vi "Conversion_from_SI_units.vi"(6 "Microsteps (MS=64)":dbl, 7 "Motor":u16(ring) items=["none", "1", "2", "3", "4", "all"], 8 "Output Unit":T1=enum."Meter", 10 "Input":dbl) -> (2 "Output":dbl)   [LabVIEW 2013]
uses:
  ConversionAndInformation/Unit_Control.ctl
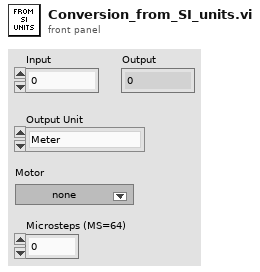
[diagram p1: front panel]
types:
  T1 = typedef "Unit_Control.ctl" = enum16{"Angle (Degrees)", "Rad", "Angle [TMC]", "Microsteps [TMC]", "Inches", "Nanometer", "Meter", "Centimeter", "Millimeter", "Micron", "Joule", "Electron Volts", "Hertz", "Terahertz", "Megahertz"}
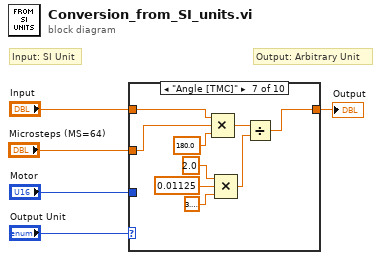
[diagram p0: block diagram]
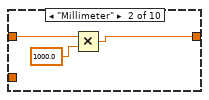
[diagram p3: hidden frame]
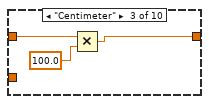
[diagram p4: hidden frame]
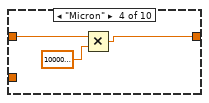
[diagram p5: hidden frame]
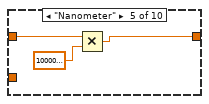
[diagram p6: hidden frame]
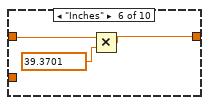
[diagram p7: hidden frame]
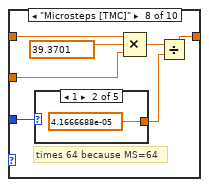
[diagram p8: hidden frame]
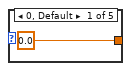
[diagram p9: hidden frame]
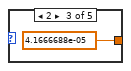
[diagram p10: hidden frame]
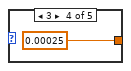
[diagram p11: hidden frame]
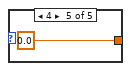
[diagram p12: hidden frame]
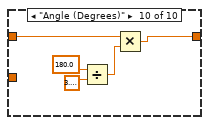
[diagram p14: hidden frame]
diagram:
  # "Output: Arbitrary Unit"
  # "Input: SI Unit"
  n1 = case shown="\"Angle [TMC]\"" "Output Unit" {
    tunnel: "Input" -> [w6 w9 w12 w15 w18 w20 w30 w35 w43 w46]
    tunnel: [w6 w8 w10 w14 w17 w19 w26 w34 w43 w44] -> w5
    tunnel: "Motor" -> [_ _ _ _ _ _ _ w33 _ _]
    tunnel: "Microsteps (MS=64)" -> [_ _ _ _ _ _ w22 w32 _ _]
    frame "Meter", Default {
    }
    frame "Millimeter" {
      n2 = Multiply(x=w9, y=1000.0) -> (x*y=w8:dbl)
    }
    frame "Centimeter" {
      n3 = Multiply(x=w12, y=100.0) -> (x*y=w10:dbl)
    }
    frame "Micron" {
      n4 = Multiply(x=w15, y=1000000.0) -> (x*y=w14:dbl)
    }
    frame "Nanometer" {
      n5 = Multiply(x=w18, y=1000000000.0) -> (x*y=w17:dbl)
    }
    frame "Inches" {
      n6 = Multiply(x=w20, y=39.3701) -> (x*y=w19:dbl)
    }
    frame "Angle [TMC]" {
      n7 = Compound Arithmetic op=MULTIPLY(w30, w22, 180.0 ("y")) -> (w28:dbl)
      n8 = Compound Arithmetic op=MULTIPLY(2.0 ("x"), 0.01125, 3.141592653589793) -> (w27:dbl)
      n9 = Divide(x=w28, y=w27) -> (x/y=w26:dbl)
    }
    frame "Microsteps [TMC]" {
      # "times 64 because MS=64"
      n10 = case shown="1" w33 {
        tunnel: [0.0 4.1666688e-05 4.1666688e-05 0.00025 0.0] -> w31
        frame 0, Default {
        }
        frame 1 {
        }
        frame 2 {
        }
        frame 3 {
        }
        frame 4 {
        }
      }
      n11 = Compound Arithmetic op=MULTIPLY(w35, 39.3701, w32) -> (w36:dbl)
      n12 = Divide(x=w36, y=w31) -> (x/y=w34:dbl)
    }
    frame "Rad" {
    }
    frame "Angle (Degrees)" {
      n13 = Divide(x=180.0 ("y"), y=3.141592653589793) -> (x/y=w45:dbl)
      n14 = Multiply(x=w46, y=w45) -> (x*y=w44:dbl)
    }
  }
  "Output" <- w5
